vi "DecodeInt16.vi"(1 "Data In":u8[](array[numeric])) -> (0 "Data Out":i16[](array[numeric]))   [LabVIEW 2015, in "navX Library v1 (deprecated).lvlib"]
uses:
  navX Library v1 (deprecated).lvlib
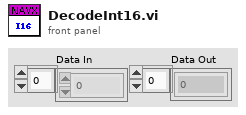
[diagram p1: front panel]
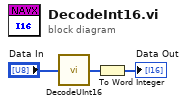
[diagram p0: block diagram]
diagram:
  n1 = call "DecodeUInt16.vi"("Data In"="Data In") -> ("Data Out"=w2:u16[])
  n2 = To Word Integer(number=w2) -> (16bit integer=→"Data Out":i16[])
